vi "FloatingMean_Example_IMAQ.vi"() -> ()   [LabVIEW 2019]
doc: "This example shows how to compute and show a floating mean live image.\nHere the camera class is operated in fifo mode to always get next image in buffer.\nThe Average Count defines the number of images that will be averaged.\nAveraging is done by fetiching one image and using average image from previous iteration\n(avg_n = (1-1/avg_count)*avg_(n-1) + (1/avg_count)*image_n)\n\nIt is a good starting point for writing own applications.\nBut it will not be fail save, i.e. doesnt react on errors, just handles them forward to the end\n\nUsage:\nSelect your required fifo buffer size and image format and start the program.\nOnce started, the camera class will be initialized and image record will start automatically.\nInside the acquisition loop the program calculates the floating average image shows it.\nThe average count can be changed at any time.\nBy using the ROI parameters you can crop the image to select certain regions\n\nBy clicking Quit Application the record will stop and will force an exit of the camera class"
uses:
  camera/Camera.lvclass
  <vilib>/vision/NI_Vision_Development_Module.lvlib
panel:
  out "nominatorU64":u64 format="%x"
  out "denominatorU64":u64 format="%x"
  out "currentImage":T1(plugin-control)
  out "nominatorU32":u64 format="%x"
  out "denominatorU32":u64 format="%x"
  in  "averageCount":u8=10 caption="Average Count" min=2
  out "Image":T1(plugin-control)
  in  "data_format":T2(ring)=enum."Mono16"
  out "Recorded Images":u32
  in  "Quit":bool
  in  "cropY1":u64=2048 min=2 max=20000 step=1
  in  "cropX1":u64=2048 min=2 max=20000 step=1
  in  "cropY0":u64=1 min=1 max=1039 step=1
  in  "cropX0":u64=1 min=1 max=1391 step=1
  out "Image Height":u64
  out "Image Width":u64
  in  "dwImgCount":u32=10 caption="Fifo Buffer Size" max=4023
  out "Error":errorcluster {"code" format="%x"}
  # "This example shows how to compute and show a floating mean live image.\nHere the camera class is operated in fifo mode to always get next image in buffer.\nThe Average Count defines the number of images that will be averaged.\nAveraging is done by fetiching one image and using average image from previous iteration\n(avg_n = (1-1/avg_count)*avg_(n-1) + (1/avg_count)*image_n)\n\nIt is a good starting point for writing own applications.\nBut it will not be fail save, i.e. doesnt react on errors, just handles them forward to the end\n\nUsage:\nSelect your required fifo buffer size and image format and start the program.\nOnce started, the camera class will be initialized and image record will start automatically.\nInside the acquisition loop the program calculates the floating average image shows it.\nThe average count can be changed at any time.\nBy using the crop parameters you can crop the image to select certain regions\n\nBy clicking Quit Application the record will stop and will force an exit of the camera class"
  # "pco.labview"
  # "Camera Setup"
  # "Recording Control"
  # "Parameters for image readout"
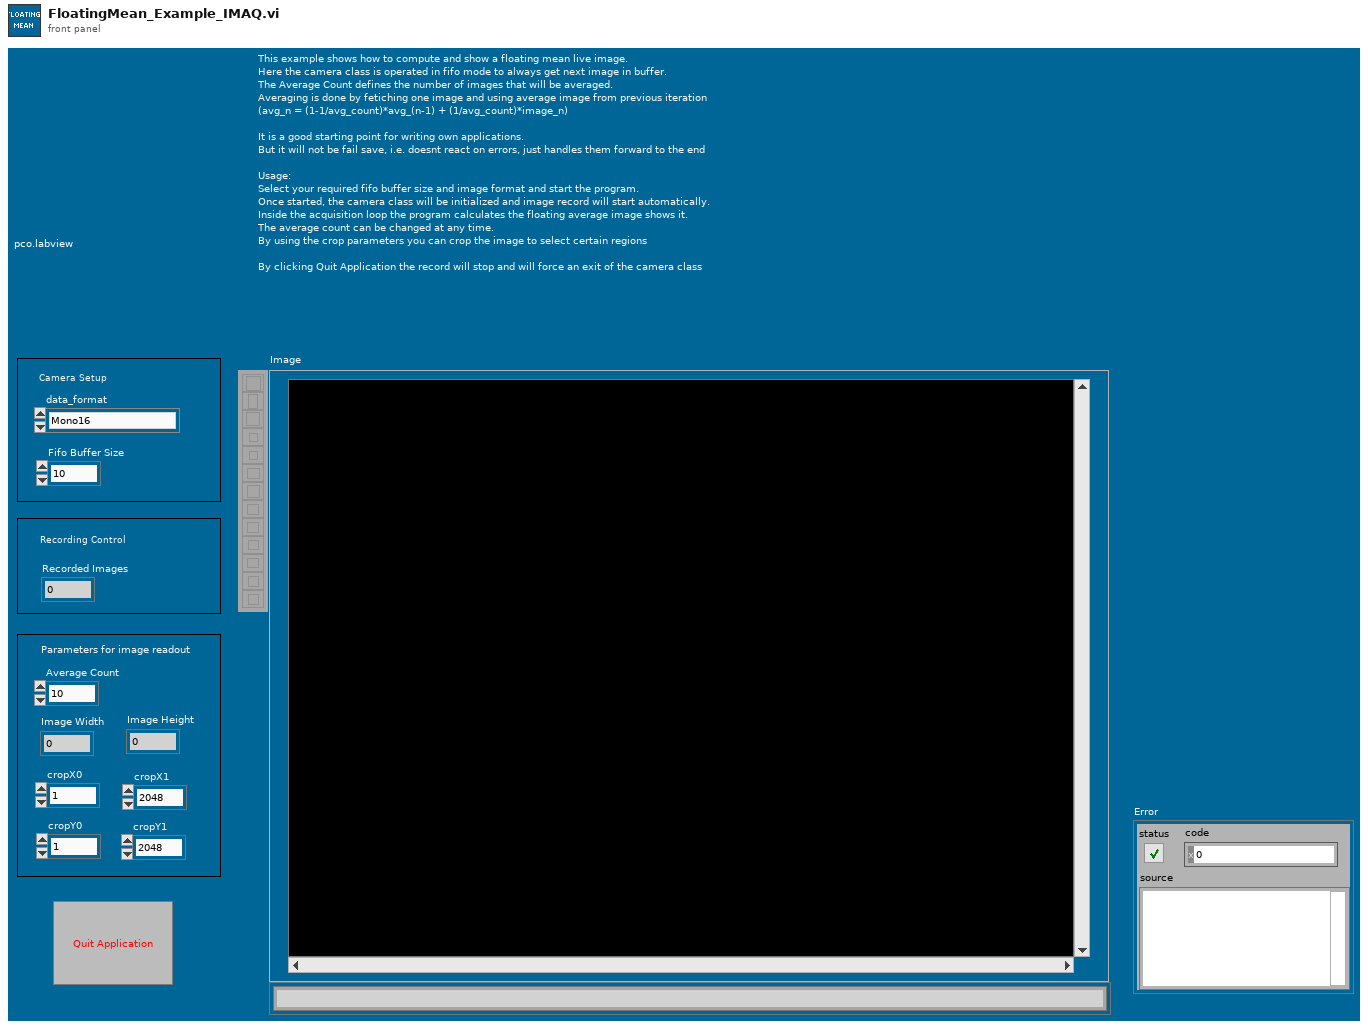
[diagram p1: front panel]
types:
  T1 = typedef "IMAQ Image.ctl" = refnum<image>
  T2 = enum16{"Undefined", "Mono8", "Mono16", "BGRA8", "RGBA8", "BGRA16", "RGBA16", "CompressedMono8"}
  T3 = enum8{"Enabled", "Disabled", "Disabled and Grayed Out"}
  T4 = enum16{"sequence", "sequence non blocking", "ring buffer", "fifo", "tif", "multitif", "pcoraw", "b16", "dicom", "multidicom", "camram_ring", "camram_segment"}
  T5 = cluster{"serial":u32, "type":u16, "sub_type":u16, "interface_type":u16, "bit_resolution":u16, "min_exposure_time_s":dbl, "max_exposure_time_s":dbl, "min_exposure_step_s":dbl, "min_delay_time_s":dbl, "max_delay_time_s":dbl, "min_delay_step_s":dbl, "min_width":u64, "min_height":u64, "max_width":u64, "max_height":u64, "roi_step_horz":u64, "roi_step_vert":u64, "roi_symmetric_horz":bool, "roi_symmetric_vert":bool, "has_timestamp_mode":bool, "has_timestamp_mode_ascii_only":bool, "pixelrate_vec":u32[], "conversion_factor_vec":sgl[], "has_trigger_mode_extexpctrl":bool, "has_acquire_mode":bool, "has_ext_acquire_mode":bool, "has_metadata_mode":bool, "has_ram":bool, "binning_horz_vec":u16[], "binning_vert_vec":u16[], "has_average_binning":bool, "pixel_format_vec":u32[]}
  T6 = typedef "Image Type" = u32
  T7 = typedef "Camera.lvclass/binning.ctl" = cluster{"vert":u16, "horz":u16, "mode":u16}
  T8 = cluster{"exposure_time_s":dbl, "delay_time_s":dbl, "roi":cluster{"x0":u64, "y0":u64, "x1":u64, "y1":u64}, "timestamp_mode":u16, "pixelrate":u32, "conversion_factor":sgl, "trigger_mode":u16, "acquire_mode":u16, "acquire_sequence_number":u32, "metadata_mode":u16, "noisefilter_mode":u16, "pixel_format":u32, "binning":T7, "auto_exposure":cluster{"region":u16, "min_exposure_s":dbl, "max_exposure_s":dbl}}
  T9 = cluster{"Plane 4 (alpha)":u16, "Plane 1 (Red)":u16, "Plane 2 (Green)":u16, "Plane 3 (Blue)":u16}[][]
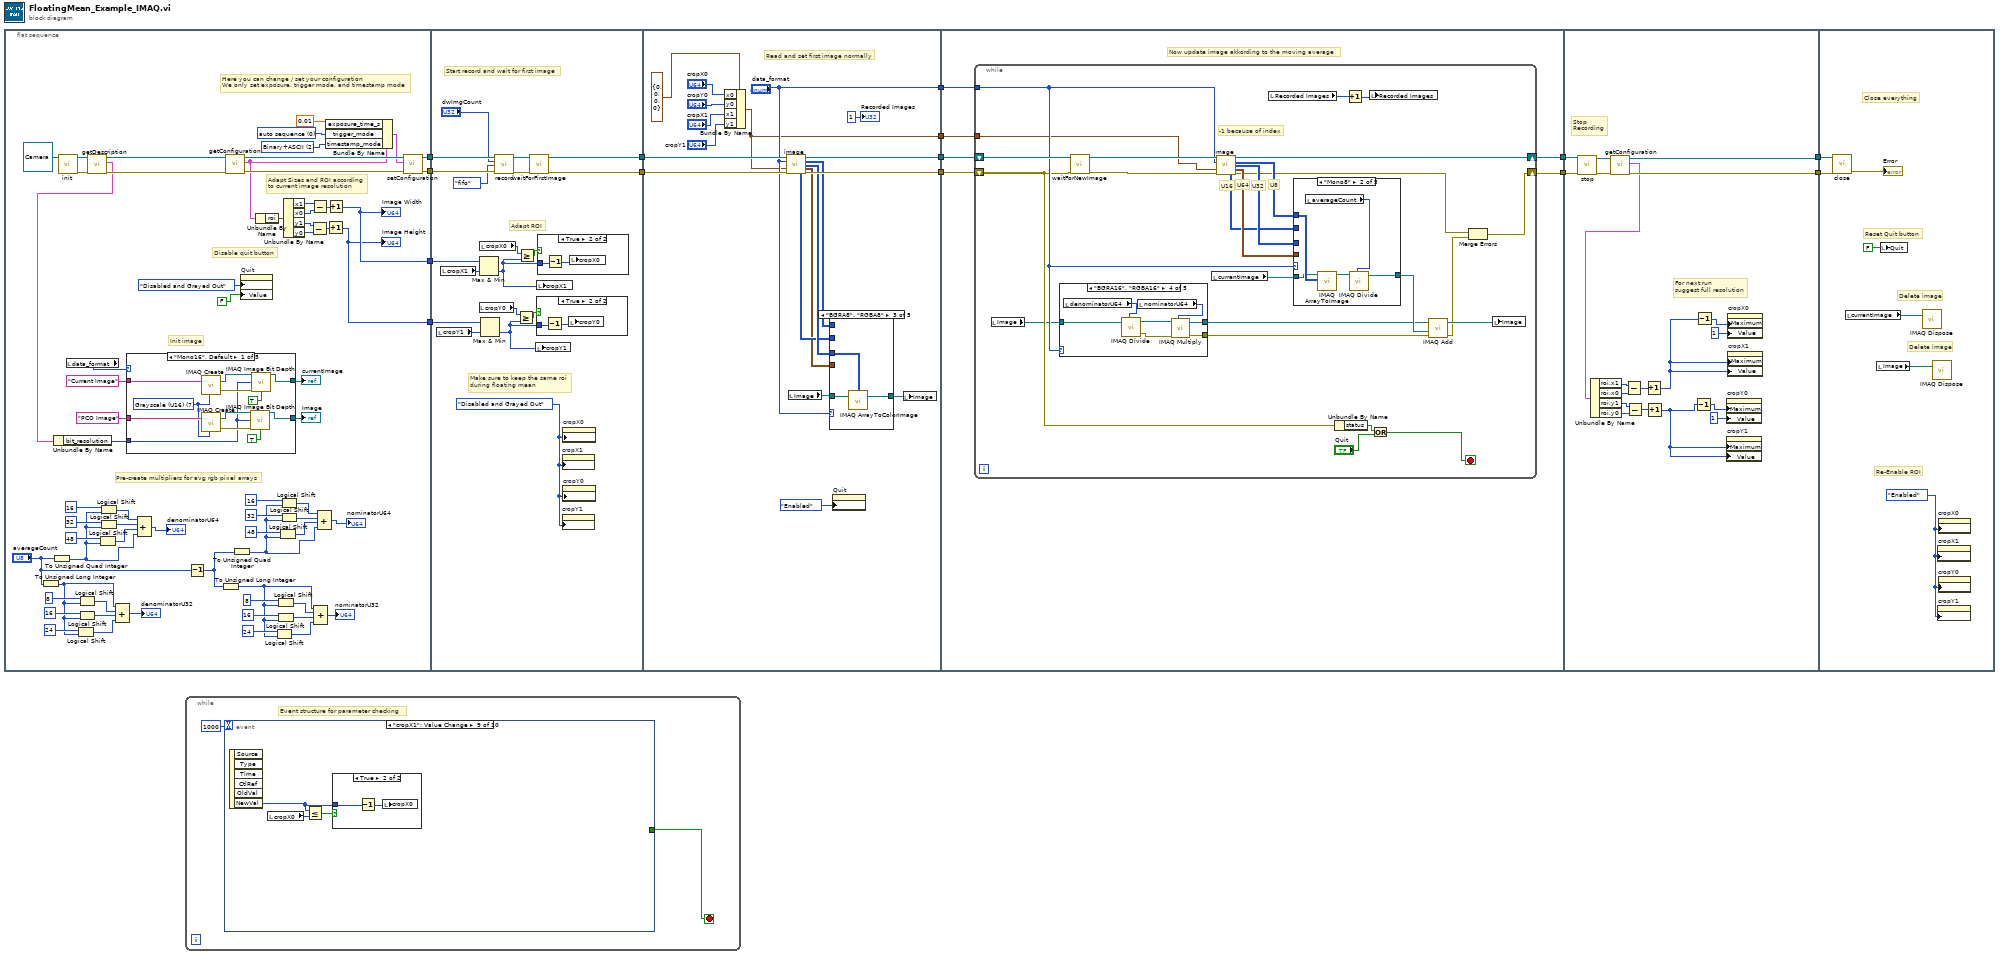
[diagram p0: block diagram]
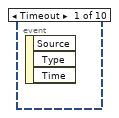
[diagram p2: hidden frame]
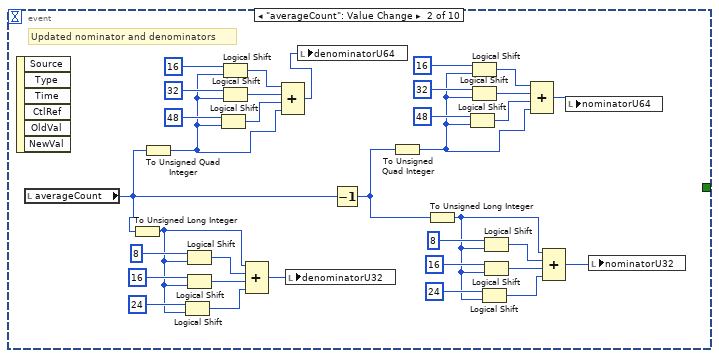
[diagram p3: hidden frame]
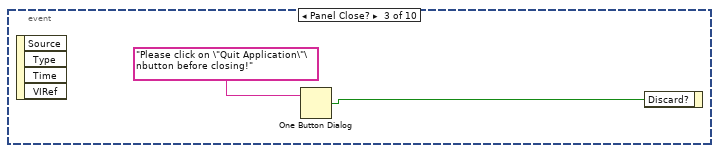
[diagram p4: hidden frame]
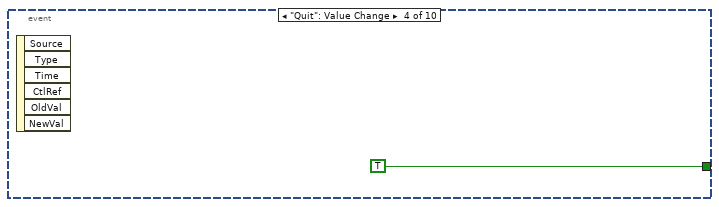
[diagram p5: hidden frame]
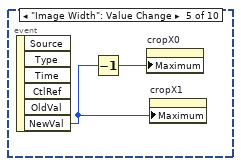
[diagram p6: hidden frame]
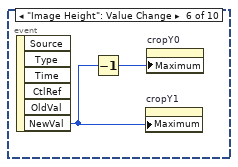
[diagram p7: hidden frame]
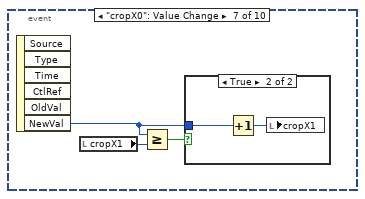
[diagram p8: hidden frame]
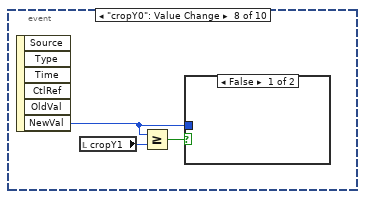
[diagram p10: hidden frame]
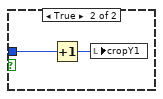
[diagram p11: hidden frame]
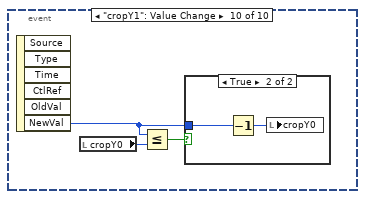
[diagram p13: hidden frame]
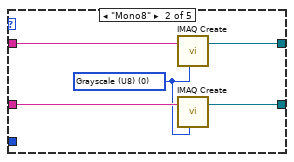
[diagram p15: hidden frame]
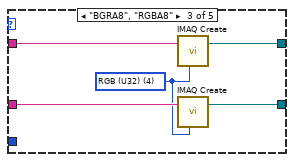
[diagram p16: hidden frame]
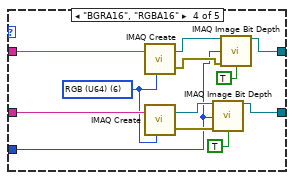
[diagram p17: hidden frame]
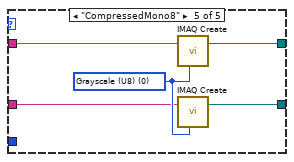
[diagram p18: hidden frame]
diagram:
  n1 = flat-sequence {
    tunnel: [w75] -> w14
    tunnel: [w74] -> w13
    tunnel: [w23] -> w2
    tunnel: [w22] -> w1
    tunnel: w14 -> [w138]
    tunnel: w13 -> [w137]
    tunnel: [w133] -> w12
    tunnel: [w132] -> w11
    tunnel: w2 -> [w129]
    tunnel: w1 -> [w127]
    tunnel: w12 -> [w160]
    tunnel: w11 -> [w159]
    tunnel: [w155] -> w10
    tunnel: [w156] -> w9
    tunnel: ["data_format"] -> w4
    tunnel: [w143] -> w3
    tunnel: w10 -> [w181]
    tunnel: w9 -> [w182]
    tunnel: [w180] -> w8
    tunnel: [w179] -> w6
    tunnel: w4 -> [w178]
    tunnel: w3 -> [w177]
    tunnel: w8 -> [w286]
    tunnel: [w281] -> w7
    tunnel: w6 -> [w285]
    tunnel: [w282] -> w5
    tunnel: w7 -> [w291]
    tunnel: w5 -> [w290]
    frame #0 {
      w65 = u16 2 items=["OFF", "Binary", "Binary+ASCII", "ASCII"] ("TimestampMode")
      w79 = u16 0 items=["auto sequence"=0, "software trigger"=1, "external exposure start & software trigger"=2, "external exposure control"=3, "external synchronized"=4, "fast external exposure control"=5, "external CDS control"=6, "slow external exposure control"=7, "external synchronized HDSDI"=258] ("TriggerMode")
      # "Here you can change / set your configuration\nWe only set exposure, trigger mode, and timestamp mode"
      # "Pre-create multipliers for avg rgb pixel arrays"
      # "Init image"
      # "Adapt Sizes and ROI according\nto current image resolution"
      # "Disable quit button"
      n2 = To Unsigned Long Integer(number="averageCount") -> (unsigned 32bit integer=w45:u32)
      n3 = To Unsigned Quad Integer(1:"averageCount") -> (0:w25:u64)
      n4 = call-dynamic "init.vi"("Camera in"=refnum<class "Camera.lvclass"> refnum ("PCOCamera in")) -> ("Camera out"=w20:refnum<class "Camera.lvclass">, "error out"=w21:errorcluster)  [unwired: 8 in]
      n5 = local read "data_format"() -> (w62:T2)
      n6 = Logical Shift(y=u32 24, x=w45) -> (x << y=w56:u32)
      n7 = Logical Shift(y=u32 8, x=w45) -> (x << y=w54:u32)
      n8 = Logical Shift(y=u32 16, x=w45) -> (x << y=w55:u32)
      n9 = call-dynamic "getDescription.vi"("error in (no error)"=w21, "Camera in"=w20) -> ("error out"=w18:errorcluster, "description"=w17:T5, "Camera out"=w19:refnum<class "Camera.lvclass">)  [unwired: 7 in]
      n10 = Unbundle By Name(w17) -> ("bit_resolution"=w16:u16)
      n11 = Logical Shift(y=u32 48, x=w25) -> (x << y=w38:u64)
      n12 = Logical Shift(y=u32 16, x=w25) -> (x << y=w36:u64)
      n13 = Logical Shift(y=u32 32, x=w25) -> (x << y=w37:u64)
      n14 = Compound Arithmetic op=ADD(w45, w54, w55, w56) -> (→"denominatorU32":u32)
      n15 = case shown="\"Mono16\", Default" w62 {
        tunnel: "PCO Image" ("Image Name") -> [w92 w95 w100 w114 w117]
        tunnel: [w86 w97 w102 w108 w119] -> w61
        tunnel: [w82 w96 w101 w105 w116] -> w43
        tunnel: "Current Image" ("Image Name") -> [w90 w94 w98 w112 w115]
        tunnel: w16 -> [w81 _ _ w103 _]
        frame "Mono16", Default {
          w91 = T6 7 items=["Grayscale (U8)", "Grayscale (I16)", "Grayscale (SGL)", "Complex (CSG)", "RGB (U32)", "HSL (U32)", "RGB (U64)", "Grayscale (U16)"] ("Image Type")
          n16 = call "IMAQ Create"("Image Name"=w90, "Image Type"=w91) -> ("New Image"=w84:T1, "error out"=w83:errorcluster)  [unwired: 3 in]
          n17 = call "IMAQ Create"("Image Name"=w92, "Image Type"=w91) -> ("New Image"=w88:T1, "error out"=w87:errorcluster)  [unwired: 3 in]
          n18 = call "IMAQ Image Bit Depth"("Image"=w88, "Bit Depth (0)"=w81, "error in (no error)"=w87, "Get/Set Bit Depth? (Set)"=TRUE) -> ("Image Out"=w86:T1)  [unwired: 9 in, 2 out]
          n19 = call "IMAQ Image Bit Depth"("Image"=w84, "Bit Depth (0)"=w81, "error in (no error)"=w83, "Get/Set Bit Depth? (Set)"=TRUE) -> ("Image Out"=w82:T1)  [unwired: 9 in, 2 out]
        }
        frame "Mono8" {
          w93 = T6 0 items=["Grayscale (U8)", "Grayscale (I16)", "Grayscale (SGL)", "Complex (CSG)", "RGB (U32)", "HSL (U32)", "RGB (U64)", "Grayscale (U16)"] ("Image Type")
          n20 = call "IMAQ Create"("Image Name"=w94, "Image Type"=w93) -> ("New Image"=w96:T1)  [unwired: 3 in, 1 out]
          n21 = call "IMAQ Create"("Image Name"=w95, "Image Type"=w93) -> ("New Image"=w97:T1)  [unwired: 3 in, 1 out]
        }
        frame "BGRA8", "RGBA8" {
          w99 = T6 4 items=["Grayscale (U8)", "Grayscale (I16)", "Grayscale (SGL)", "Complex (CSG)", "RGB (U32)", "HSL (U32)", "RGB (U64)", "Grayscale (U16)"] ("Image Type")
          n22 = call "IMAQ Create"("Image Name"=w98, "Image Type"=w99) -> ("New Image"=w101:T1)  [unwired: 3 in, 1 out]
          n23 = call "IMAQ Create"("Image Name"=w100, "Image Type"=w99) -> ("New Image"=w102:T1)  [unwired: 3 in, 1 out]
        }
        frame "BGRA16", "RGBA16" {
          w113 = T6 6 items=["Grayscale (U8)", "Grayscale (I16)", "Grayscale (SGL)", "Complex (CSG)", "RGB (U32)", "HSL (U32)", "RGB (U64)", "Grayscale (U16)"] ("Image Type")
          n24 = call "IMAQ Create"("Image Name"=w112, "Image Type"=w113) -> ("New Image"=w106:T1, "error out"=w104:errorcluster)  [unwired: 3 in]
          n25 = call "IMAQ Create"("Image Name"=w114, "Image Type"=w113) -> ("New Image"=w110:T1, "error out"=w109:errorcluster)  [unwired: 3 in]
          n26 = call "IMAQ Image Bit Depth"("Image"=w110, "Bit Depth (0)"=w103, "error in (no error)"=w109, "Get/Set Bit Depth? (Set)"=TRUE) -> ("Image Out"=w108:T1)  [unwired: 9 in, 2 out]
          n27 = call "IMAQ Image Bit Depth"("Image"=w106, "Bit Depth (0)"=w103, "error in (no error)"=w104, "Get/Set Bit Depth? (Set)"=TRUE) -> ("Image Out"=w105:T1)  [unwired: 9 in, 2 out]
        }
        frame "CompressedMono8" {
          w118 = T6 0 items=["Grayscale (U8)", "Grayscale (I16)", "Grayscale (SGL)", "Complex (CSG)", "RGB (U32)", "HSL (U32)", "RGB (U64)", "Grayscale (U16)"] ("Image Type")
          n28 = call "IMAQ Create"("Image Name"=w115, "Image Type"=w118) -> ("New Image"=w116:T1)  [unwired: 3 in, 1 out]
          n29 = call "IMAQ Create"("Image Name"=w117, "Image Type"=w118) -> ("New Image"=w119:T1)  [unwired: 3 in, 1 out]
        }
      }
      "Image" <- w61
      "currentImage" <- w43
      n30 = Compound Arithmetic op=ADD(w36, w37, w38, w25) -> (→"denominatorU64":u64)
      n31 = Decrement(x="averageCount") -> (x-1=w26:u8)
      n32 = To Unsigned Long Integer(number=w26) -> (unsigned 32bit integer=w44:u32)
      n33 = call-dynamic "getConfiguration.vi"("error in (no error)"=w18, "Camera in"=w19) -> ("error out"=w77:errorcluster, "configuration"=w73:T8, "Camera out"=w78:refnum<class "Camera.lvclass">)  [unwired: 7 in]
      n34 = To Unsigned Quad Integer(1:w26) -> (0:w24:u64)
      n35 = property on="Quit" class="Bool (strict)"("DisabledEnum"=T3."Disabled and Grayed Out" ("Disabled"), "Value"=FALSE ("Stop")) -> ()  [unwired: 2 in, 2 out]
      n36 = Unbundle By Name(w73) -> ("roi"=w72:cluster{"x0":u64, "y0":u64, "x1":u64, "y1":u64})
      n37 = Logical Shift(y=u32 24, x=w44) -> (x << y=w49:u32)
      n38 = Logical Shift(y=u32 8, x=w44) -> (x << y=w47:u32)
      n39 = Logical Shift(y=u32 16, x=w44) -> (x << y=w48:u32)
      n40 = Logical Shift(y=u32 48, x=w24) -> (x << y=w30:u64)
      n41 = Logical Shift(y=u32 16, x=w24) -> (x << y=w32:u64)
      n42 = Logical Shift(y=u32 32, x=w24) -> (x << y=w31:u64)
      n43 = Unbundle By Name(w72) -> ("x1"=w70:u64, "x0"=w71:u64, "y1"=w68:u64, "y0"=w69:u64)
      n44 = Subtract(x=w68, y=w69) -> (x-y=w66:u64)
      n45 = Subtract(x=w70, y=w71) -> (x-y=w67:u64)
      n46 = Compound Arithmetic op=ADD(w44, w47, w48, w49) -> (→"nominatorU32":u32)
      n47 = Compound Arithmetic op=ADD(w32, w31, w30, w24) -> (→"nominatorU64":u64)
      n48 = Bundle By Name(cluster=w73, "exposure_time_s"=0.01, "trigger_mode"=w79, "timestamp_mode"=w65) -> (w76:T8)
      n49 = Increment(x=w66) -> (x+1=w22:u64)
      "Image Height" <- w22
      n50 = Increment(x=w67) -> (x+1=w23:u64)
      "Image Width" <- w23
      n51 = call-dynamic "setConfiguration.vi"("error in (no error)"=w77, "configuration"=w76, "Camera in"=w78) -> ("error out"=w74:errorcluster, "Camera out"=w75:refnum<class "Camera.lvclass">)  [unwired: 7 in]
    }
    frame #1 {
      w131 = T3."Disabled and Grayed Out" ("Disabled")
      # "Adapt ROI"
      # "Make sure to keep the same roi\nduring floating mean"
      # "Start record and wait for first image"
      n52 = local read "cropY1"() -> (w128:u64)
      n53 = local read "cropX1"() -> (w130:u64)
      n54 = local read "cropY0"() -> (w122:u64)
      n55 = local read "cropX0"() -> (w126:u64)
      n56 = Max & Min(x=w129, y=w130) -> (min(x,y)=w124:u64)  [unwired: 1 out]
      n57 = Max & Min(x=w127, y=w128) -> (min(x,y)=w121:u64)  [unwired: 1 out]
      n58 = call-dynamic "record.vi"("Camera in"=w138, "num_images"="dwImgCount", "record_mode"=T4."fifo", "error in (no error)"=w137) -> ("Camera out"=w134:refnum<class "Camera.lvclass">, "error out"=w135:errorcluster)  [unwired: 10 in]
      n59 = Greater Or Equal?(x=w122, y=w121) -> (x >= y?=w123:bool)
      n60 = Greater Or Equal?(x=w126, y=w124) -> (x >= y?=w125:bool)
      n61 = call-dynamic "waitForFirstImage.vi"("error in (no error)"=w135, "Camera in"=w134) -> ("error out"=w132:errorcluster, "Camera out"=w133:refnum<class "Camera.lvclass">)  [unwired: 8 in]
      n62 = local write "cropY1"(w121) -> ()
      n63 = local write "cropX1"(w124) -> ()
      n64 = case shown="True" w123 {
        tunnel: w121 -> [_ w140]
        frame False {
        }
        frame True {
          n65 = Decrement(x=w140) -> (x-1=w139:u64)
          n66 = local write "cropY0"(w139) -> ()
        }
      }
      n67 = case shown="True" w125 {
        tunnel: w124 -> [_ w142]
        frame False {
        }
        frame True {
          n68 = Decrement(x=w142) -> (x-1=w141:u64)
          n69 = local write "cropX0"(w141) -> ()
        }
      }
      n70 = property on="cropX1" class="DigNum (strict)"("DisabledEnum"=w131) -> ()  [unwired: 2 in, 2 out]
      n71 = property on="cropY1" class="DigNum (strict)"("DisabledEnum"=w131) -> ()  [unwired: 2 in, 2 out]
      n72 = property on="cropX0" class="DigNum (strict)"("DisabledEnum"=w131) -> ()  [unwired: 2 in, 2 out]
      n73 = property on="cropY0" class="DigNum (strict)"("DisabledEnum"=w131) -> ()  [unwired: 2 in, 2 out]
    }
    frame #2 {
      # "Read and set first image normally"
      n74 = Bundle By Name(cluster=cluster{"x0":u64, "y0":u64, "x1":u64, "y1":u64} {"x0"=0, "y0"=0, "x1"=0, "y1"=0} ("roi"), "x0"="cropX0", "y0"="cropY0", "x1"="cropX1", "y1"="cropY1") -> (w143:cluster{"x0":u64, "y0":u64, "x1":u64, "y1":u64})
      n75 = call-dynamic "image.vi"("Camera in"=w160, "data_format"="data_format", "crop"=w143, "error in (no error)"=w159) -> ("Camera out"=w155:refnum<class "Camera.lvclass">, "image (U8)"=w153:u8[][], "image (U32)"=w152:u32[][], "image (U64)"=w150:T9, "raw_image (U16)"=w151:u16[][], "error out"=w156:errorcluster)  [unwired: 3 in, 3 out]
      n76 = local read "Image"() -> (w158:T1)
      n77 = case shown="\"BGRA8\", \"RGBA8\"" "data_format" {
        tunnel: w158 -> [w164 w167 w168 w173 w176]
        tunnel: [w162 w165 w170 w171 w175] -> w149
        tunnel: w150 -> [_ _ _ w172 _]
        tunnel: w152 -> [_ _ w169 _ _]
        tunnel: w153 -> [_ w166 _ _ w174]
        tunnel: w151 -> [w163 _ _ _ _]
        frame "Mono16", Default {
          n78 = call "IMAQ ArrayToImage"("Image Pixels (U16)"=w163, "Image"=w164) -> ("Image Out"=w162:T1)  [unwired: 8 in, 1 out]
        }
        frame "Mono8" {
          n79 = call "IMAQ ArrayToImage"("Image Pixels (U8)"=w166, "Image"=w167) -> ("Image Out"=w165:T1)  [unwired: 8 in, 1 out]
        }
        frame "BGRA8", "RGBA8" {
          n80 = call "IMAQ ArrayToColorImage"("Image Pixels (U32)"=w169, "Image"=w168) -> ("Image Out"=w170:T1)  [unwired: 3 in, 1 out]
        }
        frame "BGRA16", "RGBA16" {
          n81 = call "IMAQ ArrayToColorImage"("Image"=w173, "Image Pixels (U64)"=w172) -> ("Image Out"=w171:T1)  [unwired: 3 in, 1 out]
        }
        frame "CompressedMono8" {
          n82 = call "IMAQ ArrayToImage"("Image Pixels (U8)"=w174, "Image"=w176) -> ("Image Out"=w175:T1)  [unwired: 8 in, 1 out]
        }
      }
      n83 = property on="Quit" class="Bool (strict)"("DisabledEnum"=T3."Enabled" ("Disabled")) -> ()  [unwired: 2 in, 2 out]
      n84 = local write "Image"(w149) -> ()
      "Recorded Images" <- u32 1 ("Recorded Images")
    }
    frame #3 {
      # "Now update image akkording to the moving average"
      n85 = while {
        shift-right: [w207] -> w180
        shift-left: w181 -> [w206]
        shift-right: [w187] -> w179
        shift-left: w182 -> [w193]
        tunnel: w178 -> [w196]
        tunnel: w177 -> [w183]
        stop <- w190 stop-if-true
        # "-1 because of index"
        # "U64"
        # "U32"
        # "U16"
        # "U8"
        n86 = local read "Image"() -> (w186:T1)
        n87 = case shown="\"BGRA16\", \"RGBA16\"" w196 {
          tunnel: w186 -> [w211 w219 w227 w234 w240]
          tunnel: [w210 w217 w224 w233 w238] -> w184
          tunnel: [w208 w215 w222 w231 w236] -> w194
          frame "Mono16", Default {
            n88 = local read "averageCount"() -> (w213:u8)
            n89 = call "IMAQ Divide"("Image Src A"=w211, "Constant"=w213) -> ("Image Dst Out"=w214:T1, "error out"=w209:errorcluster)  [unwired: 5 in]
            n90 = Decrement(x=w213) -> (x-1=w212:u8)
            n91 = call "IMAQ Multiply"("Image Src A"=w214, "Constant"=w212, "error in (no error)"=w209) -> ("Image Dst Out"=w210:T1, "error out"=w208:errorcluster)  [unwired: 4 in]
          }
          frame "Mono8" {
            n92 = local read "averageCount"() -> (w218:u8)
            n93 = call "IMAQ Divide"("Image Src A"=w219, "Constant"=w218) -> ("Image Dst Out"=w221:T1, "error out"=w216:errorcluster)  [unwired: 5 in]
            n94 = Decrement(x=w218) -> (x-1=w220:u8)
            n95 = call "IMAQ Multiply"("Image Src A"=w221, "Constant"=w220, "error in (no error)"=w216) -> ("Image Dst Out"=w217:T1, "error out"=w215:errorcluster)  [unwired: 4 in]
          }
          frame "BGRA8", "RGBA8" {
            n96 = local read "denominatorU32"() -> (w226:u64)
            n97 = call "IMAQ Divide"("Image Src A"=w227, "Constant"=w226) -> ("Image Dst Out"=w228:T1, "error out"=w223:errorcluster)  [unwired: 5 in]
            n98 = local read "nominatorU32"() -> (w225:u64)
            n99 = call "IMAQ Multiply"("Image Src A"=w228, "Constant"=w225, "error in (no error)"=w223) -> ("Image Dst Out"=w224:T1, "error out"=w222:errorcluster)  [unwired: 4 in]
          }
          frame "BGRA16", "RGBA16" {
            n100 = local read "denominatorU64"() -> (w230:u64)
            n101 = call "IMAQ Divide"("Image Src A"=w234, "Constant"=w230) -> ("Image Dst Out"=w235:T1, "error out"=w232:errorcluster)  [unwired: 5 in]
            n102 = local read "nominatorU64"() -> (w229:u64)
            n103 = call "IMAQ Multiply"("Image Src A"=w235, "Constant"=w229, "error in (no error)"=w232) -> ("Image Dst Out"=w233:T1, "error out"=w231:errorcluster)  [unwired: 4 in]
          }
          frame "CompressedMono8" {
            n104 = local read "averageCount"() -> (w239:u8)
            n105 = call "IMAQ Divide"("Image Src A"=w240, "Constant"=w239) -> ("Image Dst Out"=w242:T1, "error out"=w237:errorcluster)  [unwired: 5 in]
            n106 = Decrement(x=w239) -> (x-1=w241:u8)
            n107 = call "IMAQ Multiply"("Image Src A"=w242, "Constant"=w241, "error in (no error)"=w237) -> ("Image Dst Out"=w238:T1, "error out"=w236:errorcluster)  [unwired: 4 in]
          }
        }
        n108 = call-dynamic "waitForNewImage.vi"("error in (no error)"=w193, "Camera in"=w206) -> ("error out"=w202:errorcluster, "Camera out"=w203:refnum<class "Camera.lvclass">)  [unwired: 8 in]
        n109 = local read "currentImage"() -> (w195:T1)
        n110 = call-dynamic "image.vi"("Camera in"=w203, "data_format"=w196, "crop"=w183, "error in (no error)"=w202) -> ("Camera out"=w207:refnum<class "Camera.lvclass">, "image (U8)"=w201:u8[][], "image (U32)"=w199:u32[][], "image (U64)"=w200:T9, "raw_image (U16)"=w198:u16[][], "error out"=w188:errorcluster)  [unwired: 3 in, 3 out]
        n111 = local read "Recorded Images"() -> (w205:u32)
        n112 = case shown="\"Mono8\"" w196 {
          tunnel: [w244 w250 w255 w260 w264] -> w185
          tunnel: w200 -> [_ _ _ w262 _]
          tunnel: w199 -> [_ _ w257 _ _]
          tunnel: w201 -> [_ w252 _ _ w267]
          tunnel: w198 -> [w247 _ _ _ _]
          tunnel: w195 -> [w243 w248 w253 w258 w263]
          frame "Mono16", Default {
            n113 = local read "averageCount"() -> (w245:u8)
            n114 = call "IMAQ ArrayToImage"("Image Pixels (U16)"=w247, "Image"=w243) -> ("Image Out"=w246:T1)  [unwired: 8 in, 1 out]
            n115 = call "IMAQ Divide"("Image Src A"=w246, "Constant"=w245) -> ("Image Dst Out"=w244:T1)  [unwired: 5 in, 1 out]
          }
          frame "Mono8" {
            n116 = local read "averageCount"() -> (w249:u8)
            n117 = call "IMAQ ArrayToImage"("Image Pixels (U8)"=w252, "Image"=w248) -> ("Image Out"=w251:T1)  [unwired: 8 in, 1 out]
            n118 = call "IMAQ Divide"("Image Src A"=w251, "Constant"=w249) -> ("Image Dst Out"=w250:T1)  [unwired: 5 in, 1 out]
          }
          frame "BGRA8", "RGBA8" {
            n119 = local read "denominatorU32"() -> (w254:u64)
            n120 = call "IMAQ ArrayToColorImage"("Image Pixels (U32)"=w257, "Image"=w253) -> ("Image Out"=w256:T1)  [unwired: 3 in, 1 out]
            n121 = call "IMAQ Divide"("Image Src A"=w256, "Constant"=w254) -> ("Image Dst Out"=w255:T1)  [unwired: 5 in, 1 out]
          }
          frame "BGRA16", "RGBA16" {
            n122 = local read "denominatorU64"() -> (w259:u64)
            n123 = call "IMAQ ArrayToColorImage"("Image"=w258, "Image Pixels (U64)"=w262) -> ("Image Out"=w261:T1)  [unwired: 3 in, 1 out]
            n124 = call "IMAQ Divide"("Image Src A"=w261, "Constant"=w259) -> ("Image Dst Out"=w260:T1)  [unwired: 5 in, 1 out]
          }
          frame "CompressedMono8" {
            n125 = local read "averageCount"() -> (w265:u8)
            n126 = call "IMAQ ArrayToImage"("Image Pixels (U8)"=w267, "Image"=w263) -> ("Image Out"=w266:T1)  [unwired: 8 in, 1 out]
            n127 = call "IMAQ Divide"("Image Src A"=w266, "Constant"=w265) -> ("Image Dst Out"=w264:T1)  [unwired: 5 in, 1 out]
          }
        }
        n128 = Unbundle By Name(w193) -> ("status"=w192:bool)
        n129 = Increment(x=w205) -> (x+1=w204:u32)
        n130 = local write "Recorded Images"(w204) -> ()
        n131 = Or(x=w192, y="Quit") -> (x .or. y?=w190:bool)
        n132 = call "IMAQ Add"("Image Src A"=w184, "Image Src B"=w185, "error in (no error)"=w194) -> ("Image Dst Out"=w197:T1, "error out"=w189:errorcluster)  [unwired: 4 in]
        n133 = Merge Errors(w188, w189) -> (w187:errorcluster)
        n134 = local write "Image"(w197) -> ()
      }
    }
    frame #4 {
      # "For next run \nsuggest full resolution"
      # "Stop \nRecording"
      n135 = call-dynamic "stop.vi"("error in (no error)"=w285, "Camera in"=w286) -> ("error out"=w283:errorcluster, "Camera out"=w284:refnum<class "Camera.lvclass">)  [unwired: 8 in]
      n136 = call-dynamic "getConfiguration.vi"("error in (no error)"=w283, "Camera in"=w284) -> ("error out"=w282:errorcluster, "configuration"=w268:T8, "Camera out"=w281:refnum<class "Camera.lvclass">)  [unwired: 7 in]
      n137 = Unbundle By Name(w268) -> ("roi.x1"=w274:u64, "roi.x0"=w273:u64, "roi.y1"=w272:u64, "roi.y0"=w271:u64)
      n138 = Subtract(x=w274, y=w273) -> (x-y=w275:u64)
      n139 = Subtract(x=w272, y=w271) -> (x-y=w276:u64)
      n140 = Increment(x=w275) -> (x+1=w279:u64)
      n141 = Increment(x=w276) -> (x+1=w278:u64)
      n142 = Decrement(x=w278) -> (x-1=w277:u64)
      n143 = Decrement(x=w279) -> (x-1=w280:u64)
      n144 = property on="cropY0" class="DigNum (strict)"("Maximum"=w277, "Value"=u64 1 ("roiY0")) -> ()  [unwired: 2 in, 2 out]
      n145 = property on="cropY1" class="DigNum (strict)"("Maximum"=w278, "Value"=w278) -> ()  [unwired: 2 in, 2 out]
      n146 = property on="cropX0" class="DigNum (strict)"("Maximum"=w280, "Value"=u64 1 ("roiX0")) -> ()  [unwired: 2 in, 2 out]
      n147 = property on="cropX1" class="DigNum (strict)"("Maximum"=w279, "Value"=w279) -> ()  [unwired: 2 in, 2 out]
    }
    frame #5 {
      w287 = T3."Enabled" ("Disabled")
      # "Re-Enable ROI"
      # "Delete image"
      # "Delete image"
      # "Reset Quit button"
      # "Close everything"
      n148 = call-dynamic "close.vi"("error in (no error)"=w290, "Camera in"=w291) -> ("error out"=→"Error":errorcluster)  [unwired: 9 in]
      n149 = local read "currentImage"() -> (w288:T1)
      n150 = local read "Image"() -> (w289:T1)
      n151 = local write "Quit"(FALSE ("Stop")) -> ()
      n152 = call "IMAQ Dispose"("Image"=w288) -> ()  [unwired: 5 in, 1 out]
      n153 = call "IMAQ Dispose"("Image"=w289) -> ()  [unwired: 5 in, 1 out]
      n154 = property on="cropX1" class="DigNum (strict)"("DisabledEnum"=w287) -> ()  [unwired: 2 in, 2 out]
      n155 = property on="cropY1" class="DigNum (strict)"("DisabledEnum"=w287) -> ()  [unwired: 2 in, 2 out]
      n156 = property on="cropX0" class="DigNum (strict)"("DisabledEnum"=w287) -> ()  [unwired: 2 in, 2 out]
      n157 = property on="cropY0" class="DigNum (strict)"("DisabledEnum"=w287) -> ()  [unwired: 2 in, 2 out]
    }
  }
  n158 = while {
    stop <- w294 stop-if-true
    # "Event structure for parameter checking"
    n159 = event shown="[8] \"cropX1\": Value Change" {
      selector: _ -> [_ _ _ _ _ _ _ _ _ _]
      dyn-events: _ -> [_ _ _ _ _ _ _ _ _ _]
      timeout: 1000 -> [_ _ _ _ _ _ _ _ _ _]
      tunnel: [_ _ _ TRUE _ _ _ _ _ _] -> w294
      event Timeout {
        n160 = event-data() -> ()  [unwired: 1 in, 3 out]
      }
      event "averageCount": Value Change {
        # "Updated nominator and denominators"
        n161 = event-data() -> ()  [unwired: 1 in, 6 out]
        n162 = local read "averageCount"() -> (w302:u8)
        n163 = To Unsigned Long Integer(number=w302) -> (unsigned 32bit integer=w315:u32)
        n164 = To Unsigned Quad Integer(1:w302) -> (0:w299:u64)
        n165 = Logical Shift(y=u32 24, x=w315) -> (x << y=w326:u32)
        n166 = Logical Shift(y=u32 8, x=w315) -> (x << y=w324:u32)
        n167 = Logical Shift(y=u32 16, x=w315) -> (x << y=w325:u32)
        n168 = Logical Shift(y=u32 48, x=w299) -> (x << y=w305:u64)
        n169 = Logical Shift(y=u32 16, x=w299) -> (x << y=w307:u64)
        n170 = Logical Shift(y=u32 32, x=w299) -> (x << y=w306:u64)
        n171 = Compound Arithmetic op=ADD(w315, w324, w325, w326) -> (w317:u32)
        n172 = Compound Arithmetic op=ADD(w307, w306, w305, w299) -> (w300:u64)
        n173 = local write "denominatorU32"(w317) -> ()
        n174 = local write "denominatorU64"(w300) -> ()
        n175 = Decrement(x=w302) -> (x-1=w308:u8)
        n176 = To Unsigned Quad Integer(1:w308) -> (0:w298:u64)
        n177 = To Unsigned Long Integer(number=w308) -> (unsigned 32bit integer=w314:u32)
        n178 = Logical Shift(y=u32 48, x=w298) -> (x << y=w311:u64)
        n179 = Logical Shift(y=u32 16, x=w298) -> (x << y=w313:u64)
        n180 = Logical Shift(y=u32 32, x=w298) -> (x << y=w312:u64)
        n181 = Logical Shift(y=u32 24, x=w314) -> (x << y=w320:u32)
        n182 = Logical Shift(y=u32 8, x=w314) -> (x << y=w318:u32)
        n183 = Logical Shift(y=u32 16, x=w314) -> (x << y=w319:u32)
        n184 = Compound Arithmetic op=ADD(w313, w312, w311, w298) -> (w301:u64)
        n185 = Compound Arithmetic op=ADD(w314, w318, w319, w320) -> (w316:u32)
        n186 = local write "nominatorU64"(w301) -> ()
        n187 = local write "nominatorU32"(w316) -> ()
      }
      event Panel Close? {
        n188 = event-data() -> ()  [unwired: 1 in, 4 out]
        n189 = One Button Dialog(message="Please click on \"Quit Application\"\nbutton before closing!") -> (true=w330:bool)  [unwired: 1 in]
        n190 = event-data("Discard?"=w330) -> ()  [unwired: 1 in, 1 out]
      }
      event "Quit": Value Change {
        n191 = event-data() -> ()  [unwired: 1 in, 6 out]
      }
      event "Image Width": Value Change {
        n192 = event-data() -> ("NewVal"=w333:u64)  [unwired: 1 in, 5 out]
        n193 = Decrement(x=w333) -> (x-1=w334:u64)
        n194 = property on="cropX0" class="DigNum (strict)"("Maximum"=w334) -> ()  [unwired: 2 in, 2 out]
        n195 = property on="cropX1" class="DigNum (strict)"("Maximum"=w333) -> ()  [unwired: 2 in, 2 out]
      }
      event "Image Height": Value Change {
        n196 = event-data() -> ("NewVal"=w335:u64)  [unwired: 1 in, 5 out]
        n197 = Decrement(x=w335) -> (x-1=w336:u64)
        n198 = property on="cropY1" class="DigNum (strict)"("Maximum"=w335) -> ()  [unwired: 2 in, 2 out]
        n199 = property on="cropY0" class="DigNum (strict)"("Maximum"=w336) -> ()  [unwired: 2 in, 2 out]
      }
      event "cropX0": Value Change {
        n200 = event-data() -> ("NewVal"=w337:u64)  [unwired: 1 in, 5 out]
        n201 = local read "cropX1"() -> (w339:u64)
        n202 = Greater Or Equal?(x=w337, y=w339) -> (x >= y?=w338:bool)
        n203 = case shown="True" w338 {
          tunnel: w337 -> [_ w341]
          frame False {
          }
          frame True {
            n204 = Increment(x=w341) -> (x+1=w340:u64)
            n205 = local write "cropX1"(w340) -> ()
          }
        }
      }
      event "cropY0": Value Change {
        n206 = event-data() -> ("NewVal"=w342:u64)  [unwired: 1 in, 5 out]
        n207 = local read "cropY1"() -> (w344:u64)
        n208 = Greater Or Equal?(x=w342, y=w344) -> (x >= y?=w343:bool)
        n209 = case shown="False" w343 {
          tunnel: w342 -> [_ w346]
          frame False {
          }
          frame True {
            n210 = Increment(x=w346) -> (x+1=w345:u64)
            n211 = local write "cropY1"(w345) -> ()
          }
        }
      }
      event "cropX1": Value Change {
        n212 = event-data() -> ("NewVal"=w347:u64)  [unwired: 1 in, 5 out]
        n213 = local read "cropX0"() -> (w349:u64)
        n214 = Less Or Equal?(x=w347, y=w349) -> (x <= y?=w348:bool)
        n215 = case shown="True" w348 {
          tunnel: w347 -> [_ w351]
          frame False {
          }
          frame True {
            n216 = Decrement(x=w351) -> (x-1=w350:u64)
            n217 = local write "cropX0"(w350) -> ()
          }
        }
      }
      event "cropY1": Value Change {
        n218 = event-data() -> ("NewVal"=w352:u64)  [unwired: 1 in, 5 out]
        n219 = local read "cropY0"() -> (w354:u64)
        n220 = Less Or Equal?(x=w352, y=w354) -> (x <= y?=w353:bool)
        n221 = case shown="True" w353 {
          tunnel: w352 -> [_ w356]
          frame False {
          }
          frame True {
            n222 = Decrement(x=w356) -> (x-1=w355:u64)
            n223 = local write "cropY0"(w355) -> ()
          }
        }
      }
    }
  }
